vi "Acq Stop.vi"(0 "session in":refnum<class "Digitizer Control.lvclass">, 1 "flush samples? (F)":bool, 5 "error in (no error)":errorcluster) -> (14 "session out":refnum<class "Digitizer Control.lvclass">, 16 "samples acquired":u64[](array[numeric]), 17 "elements to read":u64[](array[numeric]), 19 "error out":errorcluster)   [LabVIEW 2021, in "Digitizer Control.lvclass"]
doc: "Stops an acquisition.\n\nInputs:\n\n<B>session in</B>: The device session.\n\n<B>flush samples?</B>: A true on this input flushes the acquired samples. A false on this input leaves the acquired samples available for fetching.\n\nOutputs:\n\n<B>session out</B>: The device session passed on the <B>session in</B> input.\n\n<B>samples acquired</B>: The number of samples acquired since the acquisition was initiated. This output is an array, the n-th element corresponds to the n-th channel.\n\n<B>elements to read</B>: The number of elements to read from the host DMA buffer to fetch the samples acquired since the acquisition was initiated. This output is an array, the n-th element corresponds to the n-th channel."
uses:
  Digitizer Control.lvclass
  Digitizer Control.lvclass/Digitizer Control.ctl
  <vilib>/Utility/error.llb/Error Cluster From Error Code.vi
  <vilib>/rvi/interface/nirviMethod/nirviMethod.xnode
  <instrlib>/_niInstr/Streaming/v1/Host/niInstr Streaming v1 Host.lvlib
  <vilib>/FPGAPlugInAG/Dynamic/niLvFpga_StopFifo_Dynamic.vi
  <vilib>/rvi/errors/niLvFpgaMergeErrorWithErrorCode.vi
  <vilib>/FPGAPlugInAG/Dynamic/niLvFpga_StartFifo_Dynamic.vi
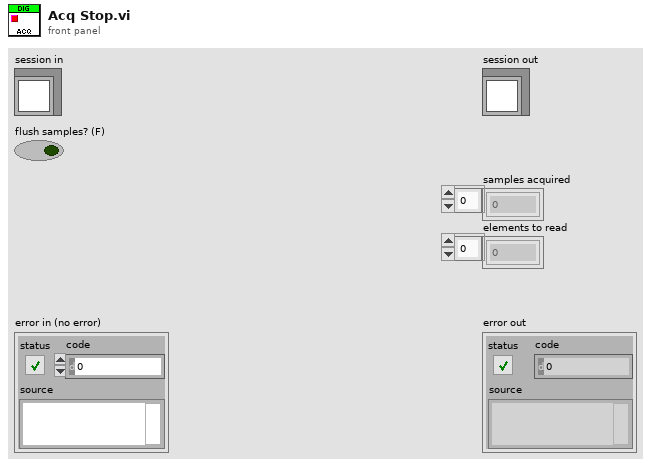
[diagram p1: front panel]
types:
  T1 = typedef "Digitizer Control.lvclass/Acq Session Data.ctl" = cluster{"ADC sampling rate":dbl, "SCTL rate":dbl, "DMA element size (bits)":i32, "sample size (bits)":i32[], "DMA/memory interface width (DMA elements)":i32, "transfer size (bits)":i32[], "stream instance":i32[], "trigger instance":u32, "group delay (s)":dbl, "data delay (s)":dbl, "target delay (s)":dbl, "trigger tracking enabled":bool, "channel configured":bool, "enabled channels":bool[], "transfer configured":bool, "dsp bypass":bool, "fractional decimator input rate":dbl, "fractional decimator output rate":dbl, "sample scale factor":dbl[], "memory size":u64[], "FIFO size":u64}
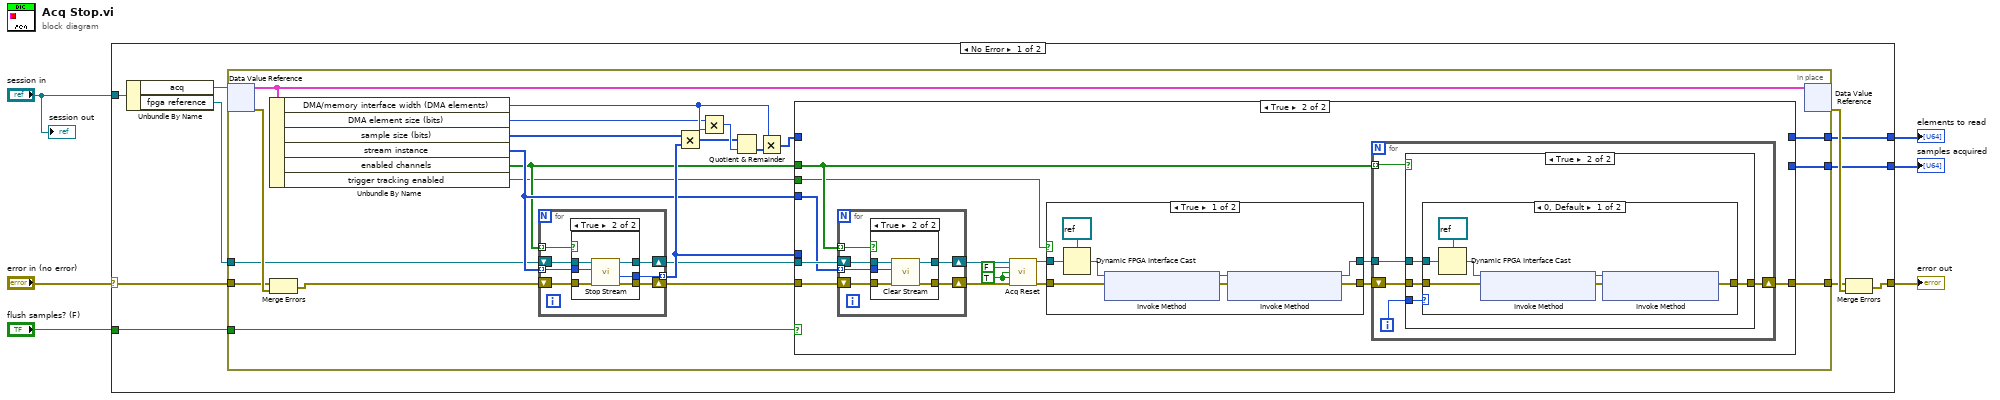
[diagram p0: block diagram]
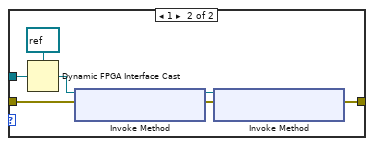
[diagram p6: hidden frame]
diagram:
  n1 = case shown="No Error" "error in (no error)" {
    selector: "error in (no error)" -> [w15 w118]
    tunnel: [w13 w118] -> w5
    tunnel: "session in" -> [w9 _]
    tunnel: [w12 _] -> w4
    tunnel: [w11 _] -> w3
    tunnel: "flush samples? (F)" -> [w10 _]
    frame No Error {
      n2 = Unbundle By Name(w9) -> ("acq"=w8:refnum<data-value>, "fpga reference"=w7:refnum<k20>)
      n3 = in-place {
        in-place-border: [w22] -> w14
        in-place-border: w15 -> [w37]
        in-place-border: [w26] -> w12
        in-place-border: [w24] -> w11
        in-place-border: w10 -> [w28]
        in-place-border: w7 -> [w19]
        n4 = in-place-dvr #1(w8) -> (w35:T1, w38:errorcluster)
        n5 = Unbundle By Name(w35) -> ("DMA/memory interface width (DMA elements)"=w30:i32, "DMA element size (bits)"=w29:i32, "sample size (bits)"=w34:i32[], "stream instance"=w20:i32[], "enabled channels"=w18:bool[], "trigger tracking enabled"=w17:bool)
        n6 = Merge Errors(w37, w38) -> (w36:errorcluster)
        n7 = for {
          tunnel: [w44] -> w27 mode=indexing
          tunnel: w20 -> [w41] mode=indexing
          shift-right: [w43] -> w23
          shift-left: w36 -> [w45]
          shift-right: [w42] -> w21
          shift-left: w19 -> [w40]
          tunnel: w18 -> [w39] mode=indexing
          n8 = case shown="True" w39 {
            tunnel: w45 -> [w46 w53]
            tunnel: [_ w52] -> w44
            tunnel: [w46 w51] -> w43
            tunnel: [w47 w50] -> w42
            tunnel: w41 -> [_ w49]
            tunnel: w40 -> [w47 w48]
            frame False {
            }
            frame True {
              n9 = call <instrlib>:"Stop Stream.vi"("error in (no error)"=w53, "stream index"=w49, "refnum in"=w48) -> ("error out"=w51:errorcluster, "samples transferred"=w52:u64, "refnum out"=w50:refnum<k20>)  [unwired: 5 in, 1 out]
            }
          }
        }
        n10 = Multiply(x=w34, y=w27) -> (x*y=w31:u64[])
        n11 = Multiply(x=w29, y=w30) -> (x*y=w33:i32)
        n12 = Quotient & Remainder(x=w31, y=w33) -> (floor(x/y)=w32:u64[])  [unwired: 1 out]
        n13 = Multiply(x=w30, y=w32) -> (x*y=w25:u64[])
        n14 = case shown="True" w28 {
          tunnel: w27 -> [w56 _]
          tunnel: [w56 _] -> w26
          tunnel: w25 -> [w55 _]
          tunnel: [w55 _] -> w24
          tunnel: w23 -> [w54 w70]
          tunnel: [w54 w63] -> w22
          tunnel: w21 -> [_ w69]
          tunnel: w20 -> [_ w68]
          tunnel: w18 -> [_ w62]
          tunnel: w17 -> [_ w61]
          frame False {
          }
          frame True {
            w64 = TRUE ("reset host streaming")
            n15 = for {
              tunnel: w68 -> [w108] mode=indexing
              shift-right: [w107] -> w67
              shift-left: w70 -> [w110]
              shift-right: [w106] -> w66
              shift-left: w69 -> [w109]
              tunnel: w62 -> [w105] mode=indexing
              n16 = case shown="True" w105 {
                tunnel: w110 -> [w111 w117]
                tunnel: w109 -> [w112 w116]
                tunnel: w108 -> [_ w115]
                tunnel: [w111 w114] -> w107
                tunnel: [w112 w113] -> w106
                frame False {
                }
                frame True {
                  n17 = call <instrlib>:"Clear Stream.vi"("error in (no error)"=w117, "stream index"=w115, "refnum in"=w116) -> ("error out"=w114:errorcluster, "refnum out"=w113:refnum<k20>)  [unwired: 7 in]
                }
              }
            }
            n18 = call "Acq Reset.vi"("fpga reference in"=w66, "reset dsp"=FALSE, "reset stream control"=w64, "reset waveform streaming"=w64, "error in (no error)"=w67) -> ("fpga reference out"=w59:refnum<k20>, "error out"=w60:errorcluster)  [unwired: 9 in]
            n19 = case shown="True" w61 {
              tunnel: w59 -> [w78 w79]
              tunnel: w60 -> [w76 w80]
              tunnel: [w72 w80] -> w57
              tunnel: [w71 w79] -> w58
              frame True {
                n20 = Dynamic FPGA Interface Cast(Session In=refnum<k20> refnum ("Type"), Type=w78) -> (Session Out=w75:refnum<k20>)
                n21 = xnode "Invoke Method"("FPGA VI Reference In"=w75, "error in"=w76) -> ("FPGA VI Reference Out"=w73:refnum<k20>, "error out"=w74:errorcluster)
                n22 = xnode "Invoke Method"("FPGA VI Reference In"=w73, "error in"=w74) -> ("FPGA VI Reference Out"=w71:refnum<k20>, "error out"=w72:errorcluster)
              }
              frame False {
              }
            }
            n23 = for {
              tunnel: w58 -> [w85]
              shift-right: [w83] -> w63
              shift-left: w57 -> [w84]
              tunnel: w62 -> [w82] mode=indexing
              i -> [w81]
              n24 = case shown="True" w82 {
                tunnel: w85 -> [_ w90]
                tunnel: w84 -> [w86 w89]
                tunnel: [w86 w88] -> w83
                tunnel: w81 -> [_ w87]
                frame False {
                }
                frame True {
                  n25 = case shown="0, Default" w87 {
                    tunnel: w90 -> [w97 w104]
                    tunnel: w89 -> [w95 w102]
                    tunnel: [w91 w98] -> w88
                    frame 0, Default {
                      n26 = Dynamic FPGA Interface Cast(Session In=refnum<k20> refnum ("Type"), Type=w97) -> (Session Out=w94:refnum<k20>)
                      n27 = xnode "Invoke Method"("FPGA VI Reference In"=w94, "error in"=w95) -> ("FPGA VI Reference Out"=w92:refnum<k20>, "error out"=w93:errorcluster)
                      n28 = xnode "Invoke Method"("FPGA VI Reference In"=w92, "error in"=w93) -> ("error out"=w91:errorcluster)  [unwired: 1 out]
                    }
                    frame 1 {
                      n29 = Dynamic FPGA Interface Cast(Session In=refnum<k20> refnum ("Type"), Type=w104) -> (Session Out=w101:refnum<k20>)
                      n30 = xnode "Invoke Method"("FPGA VI Reference In"=w101, "error in"=w102) -> ("FPGA VI Reference Out"=w99:refnum<k20>, "error out"=w100:errorcluster)
                      n31 = xnode "Invoke Method"("FPGA VI Reference In"=w99, "error in"=w100) -> ("error out"=w98:errorcluster)  [unwired: 1 out]
                    }
                  }
                }
              }
            }
          }
        }
        n32 = in-place-dvr #1(w35) -> (w16:errorcluster)  [unwired: 1 out]
      }
      n33 = Merge Errors(w14, w16) -> (w13:errorcluster)
    }
    frame Error {
    }
  }
  "error out" <- w5
  "elements to read" <- w3
  "samples acquired" <- w4
  "session out" <- "session in"
